vi "Report.vi"(6 "文件重命名":bool, 7 "文件名称":string, 8 "错误输入（无错误）":errorcluster, 11 "检测结果":bool[][](array[boolean])=[[TRUE]]) -> (0 "error out":errorcluster caption="错误输出", 3 "PRODUCT_VAULE":string)   [LabVIEW 2020]
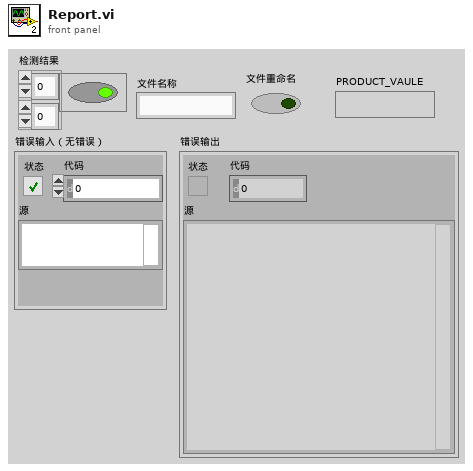
[diagram p1: front panel]
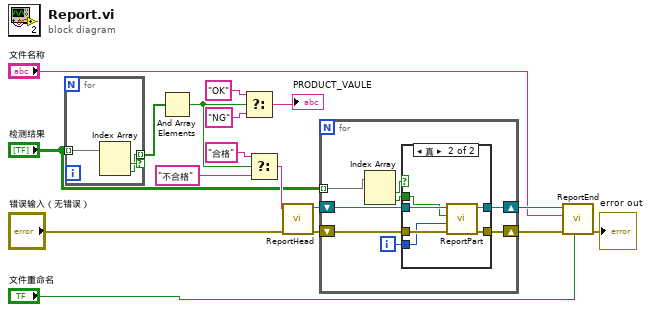
[diagram p0: block diagram]
diagram:
  n1 = for {
    tunnel: [w18] -> w3 mode=indexing if=w19
    tunnel: "检测结果" -> [w20] mode=indexing
    n2 = Index Array(array=w20) -> (element #1=w19:bool, element #2=w18:bool)  [unwired: 2 in]
  }
  n3 = And Array Elements(Boolean array=w3) -> (logical AND=w4:bool)
  n4 = Select(t="OK", s=w4, f="NG") -> (s? t:f=→"PRODUCT_VAULE":string)
  n5 = Select(t="合格", s=w4, f="不合格") -> (s? t:f=w8:string)
  n6 = call "ReportHead.vi"("error in (no error)"="错误输入（无错误）", "产品状态"=w8) -> ("error out"=w16:errorcluster, "report out"=w17:refnum<class "NI_report.lvclass">)  [unwired: 8 in]
  n7 = for {
    shift-right: [w26] -> w15
    shift-left: w17 -> [w28]
    shift-right: [w25] -> w14
    shift-left: w16 -> [w27]
    tunnel: "检测结果" -> [w23] mode=indexing
    i -> [w24]
    n8 = Index Array(array=w23) -> (element #1=w22:bool, element #2=w21:bool)  [unwired: 2 in]
    n9 = case shown="真" w22 {
      tunnel: w28 -> [w29 w36]
      tunnel: w27 -> [w30 w35]
      tunnel: [w29 w34] -> w26
      tunnel: [w30 w33] -> w25
      tunnel: w24 -> [_ w31]
      tunnel: w21 -> [_ w32]
      frame False {
      }
      frame True {
        n10 = call "ReportPart.vi"("error in"=w35, "索引"=w31, "合格"=w32, "report in"=w36) -> ("error out 2"=w33:errorcluster, "report out"=w34:refnum<class "NI_report.lvclass">)  [unwired: 6 in]
      }
    }
  }
  n11 = call "ReportEnd.vi"("文件重命名"="文件重命名", "error in (no error)"=w14, "文件名称"="文件名称", "report in"=w15) -> ("error out"=→"error out":errorcluster)  [unwired: 7 in]
